vi "send mail from computer.vi"() -> ()   [LabVIEW 2012, in "Sendmail.lvrbt"]
uses:
  Sendmail.lvrbt
  <vilib>/NXT/Block Support/NXT_MessageMailbox.ctl
  <vilib>/NXT/Block Support/NXT_InputPort.ctl
panel:
  out "String 4":string
  out "String 3":string
  out "String 2":string
  out "String":string
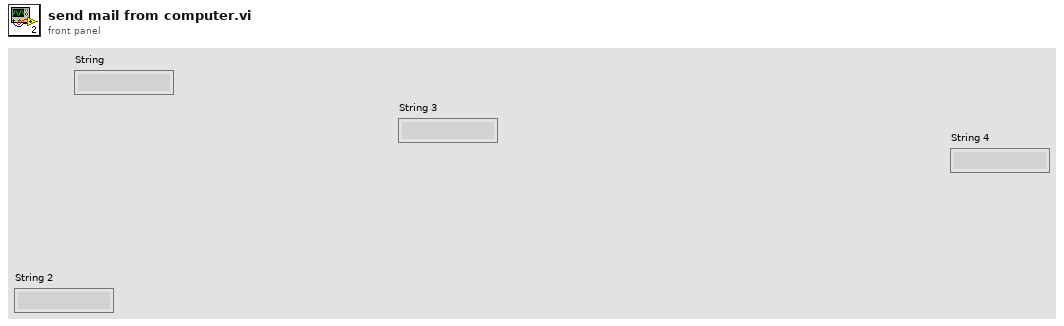
[diagram p1: front panel]
types:
  T1 = typedef "NXT_InputPort.ctl" = u8
  T2 = typedef "NXT_MessageMailbox.ctl" = u8
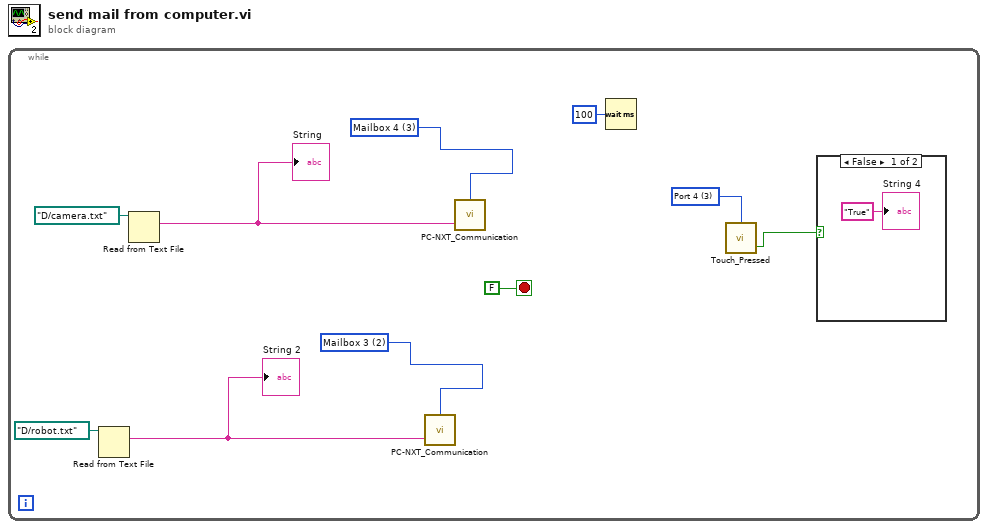
[diagram p0: block diagram]
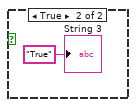
[diagram p2: hidden frame]
diagram:
  n1 = while {
    stop <- FALSE stop-if-true
    w2 = T1 3 items=["Port 1", "Port 2", "Port 3", "Port 4"] ("Port (Port 1)")
    w4 = T2 2 items=["Mailbox 1", "Mailbox 2", "Mailbox 3", "Mailbox 4", "Mailbox 5", "Mailbox 6", "Mailbox 7", "Mailbox 8", "Mailbox 9", "Mailbox 10"] ("Mailbox")
    w8 = T2 3 items=["Mailbox 1", "Mailbox 2", "Mailbox 3", "Mailbox 4", "Mailbox 5", "Mailbox 6", "Mailbox 7", "Mailbox 8", "Mailbox 9", "Mailbox 10"] ("Mailbox")
    n2 = Read from Text File(file (use dialog)=path "D:/robot.txt") -> (text=w3:string)  [unwired: 3 in, 3 out]
    "String 2" <- w3
    n3 = Read from Text File(file (use dialog)=path "D:/camera.txt") -> (text=w6:string)  [unwired: 3 in, 3 out]
    "String" <- w6
    n4 = call <vilib>:"PC-NXT_Communication.vi"("Message"=w3, "Mailbox (Mailbox 1)"=w4) -> ()  [unwired: 2 in, 1 out]
    n5 = call <vilib>:"PC-NXT_Communication.vi"("Message"=w6, "Mailbox (Mailbox 1)"=w8) -> ()  [unwired: 2 in, 1 out]
    n6 = Wait (ms)(milliseconds to wait=u32 100) -> ()  [unwired: 1 out]
    n7 = call <vilib>:"Touch_Pressed.vi"("Port (Port 1)"=w2) -> ("Yes / No"=w1:bool)  [unwired: 2 in, 1 out]
    n8 = case shown="False" w1 {
      frame False {
        "String 4" <- "True" ("String 3")
      }
      frame True {
        "String 3" <- "True" ("String 3")
      }
    }
  }
